vi "UpdateFrontPanel.vi"(0 "operation":enum16{"set references", "update"}(ring), 1 "Image Settings":refnum<vi>, 2 "Regular Controls":refnum<vi>[](array[refnum]), 3 "Special Controls":refnum<vi>[](array[refnum]), 4 "Current Position (µm)":refnum<vi>, 5 "Scan":bool) -> ()   [LabVIEW 2009]
uses:
  ImageSettings.ctt
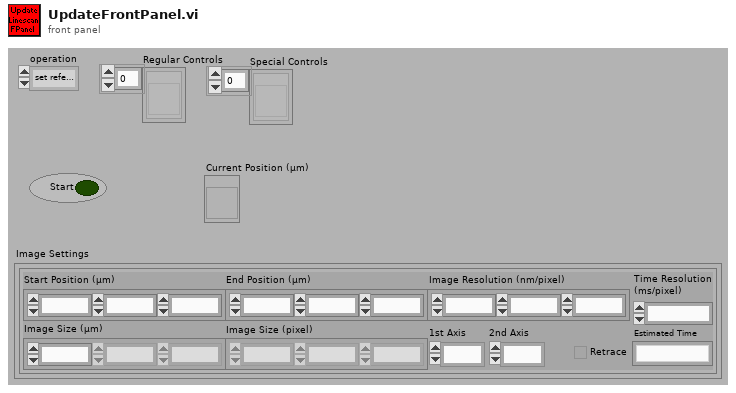
[diagram p1: front panel]
types:
  T1 = cluster{"Start Position (µm)":cluster{"x":dbl, "y":dbl, "z":dbl}, "End Position (µm)":cluster{"x":dbl, "y":dbl, "z":dbl}, "Image Resolution (nm/pixel)":cluster{"x":dbl, "y":dbl, "z":dbl}, "Image Size (µm)":cluster{"x":dbl, "y":dbl, "z":dbl}, "Image Size (pixel)":cluster{"x":u32, "y":u32, "z":u32}, "Time Resolution\n(ms/pixel)":dbl, "1st Axis":u16, "2nd Axis":u16, "Retrace":bool, "Estimated Time":string}
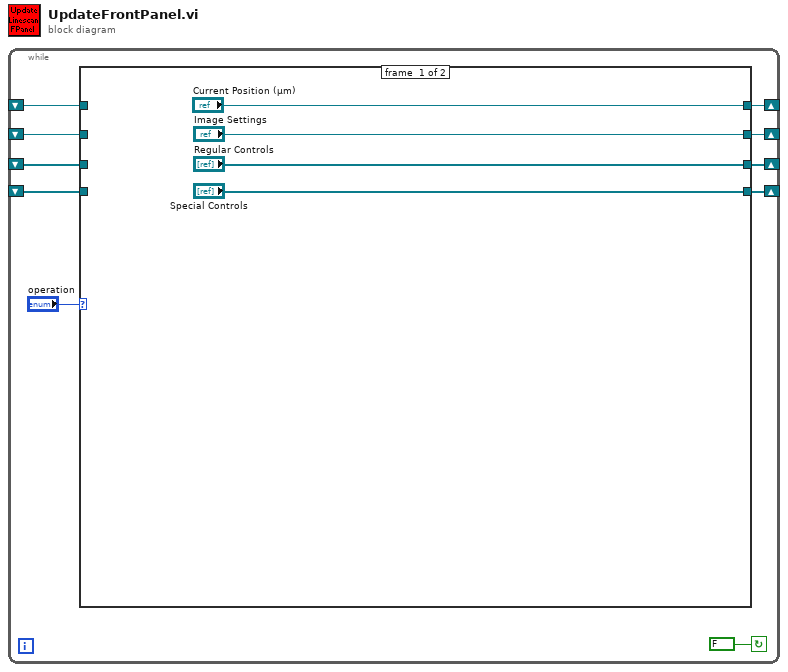
[diagram p0: block diagram]
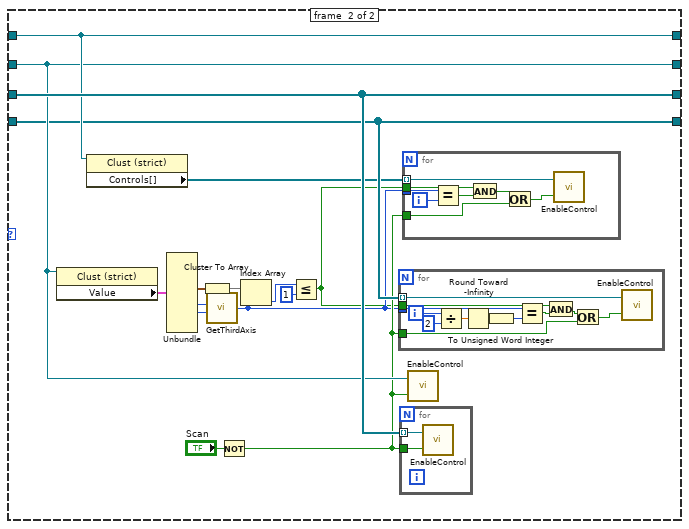
[diagram p2: hidden frame]
diagram:
  n1 = while {
    shift-right: [w8] -> _
    shift-left: _ -> [w6]
    shift-right: [w7] -> _
    shift-left: _ -> [w5]
    shift-right: [w4] -> _
    shift-left: _ -> [w3]
    shift-right: [w2] -> _
    shift-left: _ -> [w1]
    stop <- FALSE continue-if-true
    n2 = case shown="\"set references\", Default" "operation" {
      tunnel: ["Regular Controls" w30] -> w8
      tunnel: ["Special Controls" w23] -> w7
      tunnel: w6 -> [_ w30]
      tunnel: w5 -> [_ w23]
      tunnel: ["Image Settings" w27] -> w4
      tunnel: w3 -> [_ w27]
      tunnel: ["Current Position (µm)" w28] -> w2
      tunnel: w1 -> [_ w28]
      frame #0 {
      }
      frame #1 {
        n3 = property class="Clust (strict)"(reference=w27) -> ("Value"=w26:T1)  [unwired: 1 in, 2 out]
        n4 = property class="Clust (strict)"(reference=w28) -> ("Controls[]"=w22:refnum<vi>[])  [unwired: 1 in, 2 out]
        n5 = Unbundle(w26) -> ("Image Size (pixel)"=w20:cluster{"x":u32, "y":u32, "z":u32}, "1st Axis"=w25:u16, "2nd Axis"=w24:u16)  [unwired: 7 out]
        n6 = Cluster To Array(cluster=w20) -> (array=w18:u32[])
        n7 = call "GetThirdAxis.vi"("1st Axis"=w24, "2nd Axis"=w25) -> ("3rd Axis"=w19:i32)  [unwired: 2 in]
        n8 = Not(x="Scan") -> (.not. x?=w21:bool)
        n9 = Index Array(array=w18, index=w19) -> (element=w17:u32)
        n10 = Less Or Equal?(x=w17, y=u32 1) -> (x <= y?=w15:bool)
        n11 = for {
          tunnel: w23 -> [w50] mode=indexing
          tunnel: w21 -> [w43]
          tunnel: w19 -> [w45]
          tunnel: w15 -> [w39]
          i -> [w49]
          n12 = Divide(x=w49, y=2) -> (x/y=w47:dbl)
          n13 = Round Toward -Infinity(1:w47) -> (0:w46:dbl)
          n14 = To Unsigned Word Integer(number=w46) -> (unsigned 16bit integer=w44:u16)
          n15 = Equal?(x=w45, y=w44) -> (x = y?=w41:bool)
          n16 = And(x=w39, y=w41) -> (x .and. y?=w40:bool)
          n17 = Or(x=w40, y=w43) -> (x .or. y?=w42:bool)
          n18 = call "EnableControl.vi"("Enable"=w42, "Reference"=w50) -> ()
        }
        n19 = for {
          tunnel: w30 -> [w51] mode=indexing
          tunnel: w21 -> [w52]
          n20 = call "EnableControl.vi"("Enable"=w52, "Reference"=w51) -> ()
        }
        n21 = for {
          tunnel: w22 -> [w38] mode=indexing
          tunnel: w21 -> [w36]
          tunnel: w19 -> [w37]
          tunnel: w15 -> [w31]
          i -> [w34]
          n22 = Equal?(x=w37, y=w34) -> (x = y?=w33:bool)
          n23 = And(x=w31, y=w33) -> (x .and. y?=w32:bool)
          n24 = Or(x=w32, y=w36) -> (x .or. y?=w35:bool)
          n25 = call "EnableControl.vi"("Enable"=w35, "Reference"=w38) -> ()
        }
        n26 = call "EnableControl.vi"("Enable"=w21, "Reference"=w27) -> ()
      }
    }
  }
